vi "HH_PI_PhysikInstrumenteInitialisiation.vi"(8 "error in (no error)":errorcluster, 11 "PI SystemNumber":i32=1) -> (0 "error out":errorcluster, 3 "Device List":T1(array[cluster]), 5 "y-position":dbl, 6 "z-position":dbl, 7 "x-position":dbl)   [LabVIEW 2010]
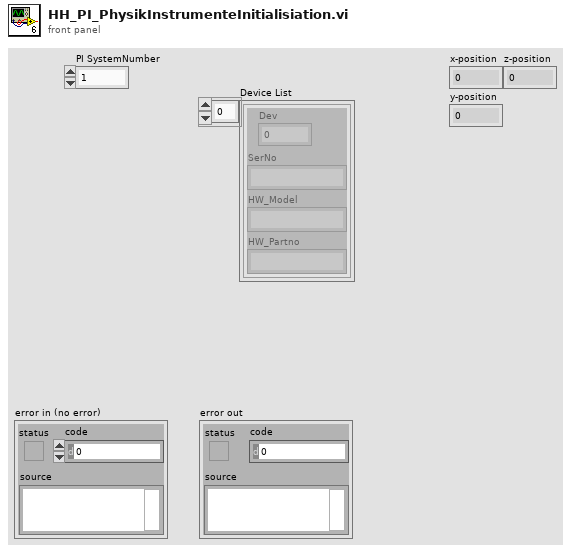
[diagram p1: front panel]
types:
  T1 = cluster{"Dev":i32, "SerNo":string, "HW_Model":string, "HW_Partno":string}[]
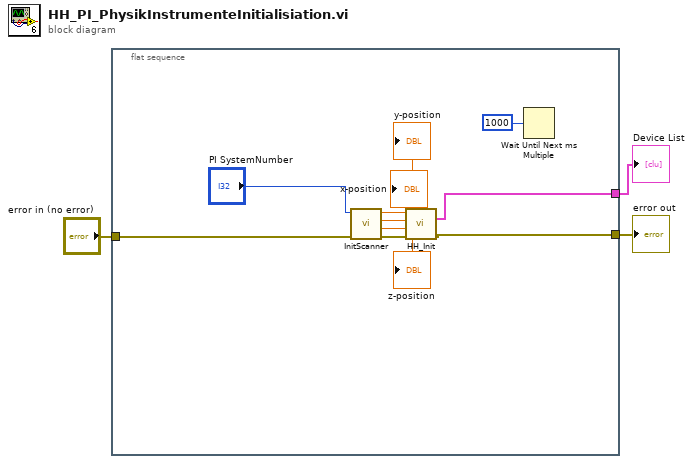
[diagram p0: block diagram]
diagram:
  n1 = flat-sequence {
    tunnel: [w12] -> w1
    tunnel: "error in (no error)" -> [w8]
    tunnel: [w9] -> w3
    frame #0 {
      n2 = call "InitScanner.vi"("error in"=w8, "PI SystemNumber"="PI SystemNumber") -> ("error out"=w11:errorcluster, "z-position"=→"z-position":dbl, "y-position"=→"y-position":dbl, "x-position"=→"x-position":dbl)  [unwired: 6 in]
      n3 = call "HH_Init.vi"("error in (no error)"=w11) -> ("Device List"=w12:T1, "error out"=w9:errorcluster)  [unwired: 12 in, 1 out]
      n4 = Wait Until Next ms Multiple(millisecond multiple=u32 1000) -> ()  [unwired: 1 out]
    }
  }
  "error out" <- w3
  "Device List" <- w1
